vi "SetParam.vi"(8 "error in (no error)":errorcluster caption="entrée d'erreur (pas d'erreur)", 10 "extract_patches_2d":T1={"patch_size"={"patch_height"=0, "patch_width"=0}, "max_patches"="None", "random_state"=-1} {"random_state" min=-1}, 11 "Extract_Patches_2d.lvclass":refnum<class "Extract_Patches_2d.lvclass">) -> (0 "error out":errorcluster caption="sortie d'erreur", 3 "Extract_Patches_2d.lvclass":refnum<class "Extract_Patches_2d.lvclass">)   [LabVIEW 2020, in "Extract_Patches_2d.lvclass"]
doc: "Set Parameters"
uses:
  Extract_Patches_2d.lvclass
  Extract_Patches_2d.lvclass/Extract_Patches_2d.ctl
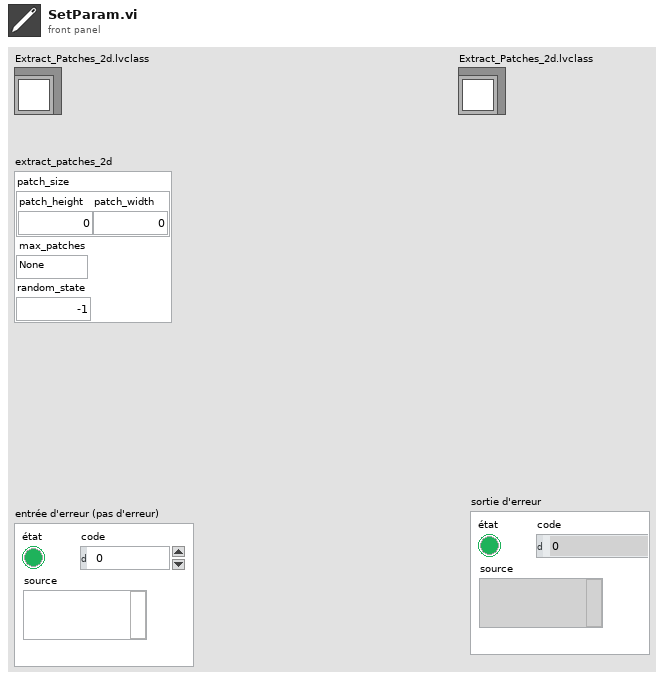
[diagram p1: front panel]
types:
  T1 = cluster{"patch_size":cluster{"patch_height":i32, "patch_width":i32}, "max_patches":string, "random_state":i32}
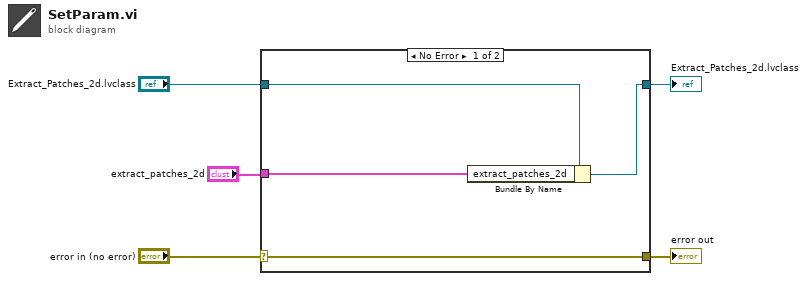
[diagram p0: block diagram]
diagram:
  n1 = case shown="No Error" "error in (no error)" {
    selector: "error in (no error)" -> [w9 w10]
    tunnel: [w9 w10] -> w4
    tunnel: [w7 w11] -> w2
    tunnel: "Extract_Patches_2d.lvclass" -> [w8 w11]
    tunnel: "extract_patches_2d" -> [w6 _]
    frame No Error {
      n2 = Bundle By Name(cluster=w8, "extract_patches_2d"=w6) -> (w7:refnum<class "Extract_Patches_2d.lvclass">)
    }
    frame Error {
    }
  }
  "error out" <- w4
  "Extract_Patches_2d.lvclass" <- w2
